vi "Get Cluster Id.vi"(8 "error in (no error)":errorcluster) -> (0 "error out":errorcluster, 3 "cluster id":string)   [LabVIEW 2021, in "NI Discovery V1 Client.lvlib"]
doc: "Advanced use only. Gets the Cluster Id which causes the next discovery client created to refer to a custom discovery service with the given id. This isolates the services launched through the discovery client to that instance."
uses:
  NI Discovery V1 Client.lvlib
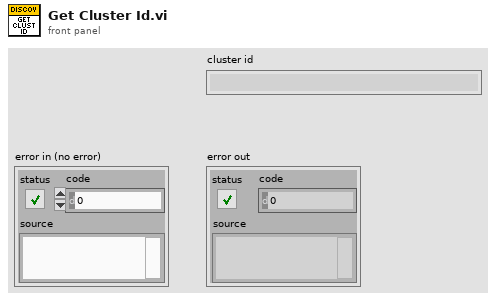
[diagram p1: front panel]
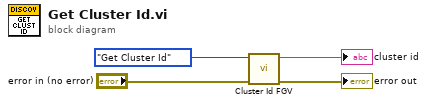
[diagram p0: block diagram]
diagram:
  n1 = call "Cluster Id FGV.vi"("error in (no error)"="error in (no error)", "action"=enum16{"Get Cluster Id", "Set Cluster Id"}."Get Cluster Id") -> ("error out"=→"error out":errorcluster, "cluster id out"=→"cluster id":string)  [unwired: 8 in]
